vi "DO线性系数设置.vi"() -> ()   [LabVIEW 2016, in "斯坦道多参数.lvlib"]
panel:
  in  "Close":bool
  in  "b":dbl format="%#.4f"
  in  "K":dbl format="%#.4f"
  in  "启用":bool
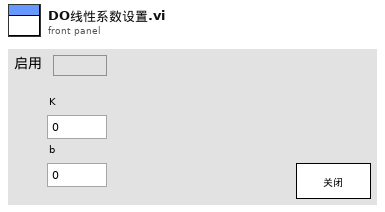
[diagram p1: front panel]
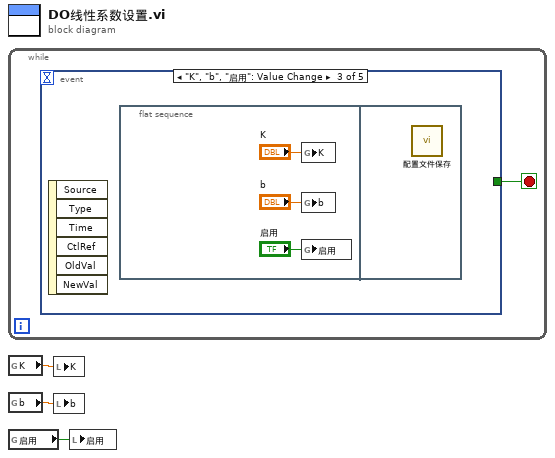
[diagram p0: block diagram]
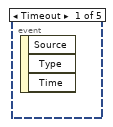
[diagram p2: hidden frame]
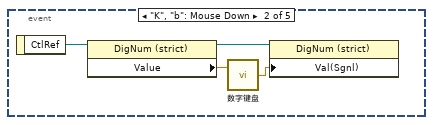
[diagram p3: hidden frame]
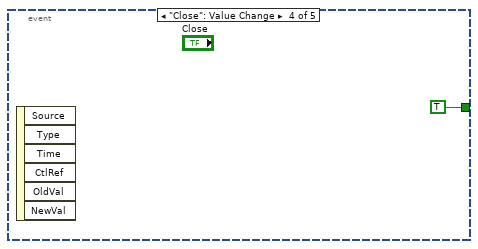
[diagram p4: hidden frame]
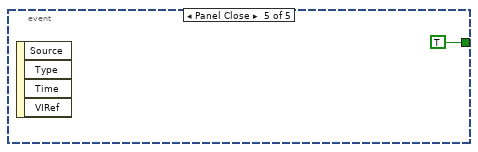
[diagram p5: hidden frame]
diagram:
  n1 = while {
    stop <- w4 stop-if-true
    n2 = event shown="[2] \"K\", \"b\", \"启用\": Value Change" {
      selector: _ -> [_ _ _ _ _]
      dyn-events: _ -> [_ _ _ _ _]
      timeout: _ -> [_ _ _ _ _]
      tunnel: [_ _ _ TRUE TRUE] -> w4
      event Timeout {
        n3 = event-data() -> ()  [unwired: 1 in, 3 out]
      }
      event "K", "b": Mouse Down {
        n4 = event-data() -> ("CtlRef"=w8:refnum<vi>)  [unwired: 1 in]
        n5 = property class="DigNum (strict)"(reference=w8) -> (reference out=w6:refnum<vi>, "Value"=w7:dbl)  [unwired: 1 in, 1 out]
        n6 = call "数字键盘.vi"("OldNumber"=w7) -> ("NewNumber"=w5:dbl)  [unwired: 1 in]
        n7 = property class="DigNum (strict)"(reference=w6, "Val(Sgnl)"=w5) -> ()  [unwired: 1 in, 2 out]
      }
      event "K", "b", "启用": Value Change {
        n8 = event-data() -> ()  [unwired: 1 in, 6 out]
        n9 = flat-sequence {
          frame #0 {
            n10 = global write "断电保存变量.vi" "K"("K") -> ()
            n11 = global write "断电保存变量.vi" "b"("b") -> ()
            n12 = global write "断电保存变量.vi" "启用"("启用") -> ()
          }
          frame #1 {
            n13 = call "配置文件保存.vi"() -> ()  [unwired: 12 in]
          }
        }
      }
      event "Close": Value Change {
        n14 = event-data() -> ()  [unwired: 1 in, 6 out]
      }
      event Panel Close {
        n15 = event-data() -> ()  [unwired: 1 in, 4 out]
      }
    }
  }
  n16 = global read "断电保存变量.vi" "K"() -> (w3:dbl)
  n17 = global read "断电保存变量.vi" "b"() -> (w2:dbl)
  n18 = global read "断电保存变量.vi" "启用"() -> (w1:bool)
  n19 = local write "K"(w3) -> ()
  n20 = local write "b"(w2) -> ()
  n21 = local write "启用"(w1) -> ()
